vi "Broadcast on FPGA IO.vi"(3 "FPGA I/O":refnum<k21>, 6 "signal in":bool, 7 "master":bool) -> (1 "signal out":bool)   [LabVIEW 2012, in "ni579x Synchronization v1 FPGA.lvlib"]
doc: "This VI takes in a signal and will broadcast it out on an FPGA I/O line IFF the master. All devices will also read this FPGA I/O line (in order to acheive the broadcast functionality). This is an opt-in design; all FPGAs need to use the same FGPA I/O line to send/receive broadcasts."
uses:
  <instrlib>/ni579x/Synchronization/v1/FPGA/ni579x Synchronization v1 FPGA.lvlib
  <vilib>/rvi/eio/common/nirviEmuTemplateMethod_errors.vi
  <vilib>/eio/EIONode/EIONode.xnode
  <vilib>/eio/EIOMethodNode/EIOMethodNode.xnode
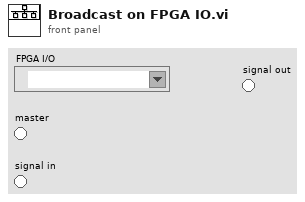
[diagram p1: front panel]
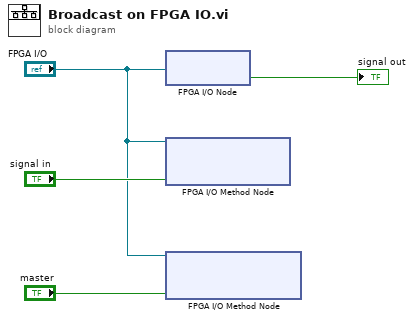
[diagram p0: block diagram]
diagram:
  n1 = xnode "FPGA I/O Node"("FPGA I/O In"="FPGA I/O") -> ("I/O Item"=→"signal out":bool)  [unwired: 1 out]
  n2 = xnode "FPGA I/O Method Node"("FPGA I/O In"="FPGA I/O", "Data"="signal in") -> ()  [unwired: 1 out]
  n3 = xnode "FPGA I/O Method Node"("FPGA I/O In"="FPGA I/O", "Enable"="master") -> ()  [unwired: 1 out]
